vi "Test phi_offset Cpp.vi"() -> ()   [LabVIEW 2011]
uses:
  gVision.lvlib
panel:
  in  "yaw":dbl
  in  "roll":dbl
  in  "pitch":dbl
  out "phi":dbl
  out "error out":errorcluster
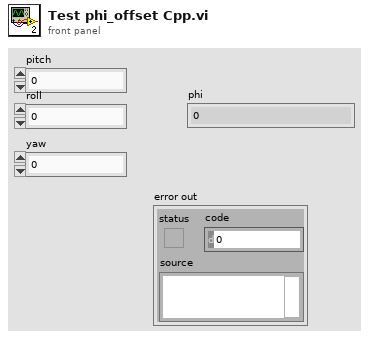
[diagram p1: front panel]
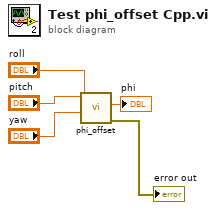
[diagram p0: block diagram]
diagram:
  n1 = call "phi_offset.vi"("yaw"="yaw", "roll"="roll", "pitch"="pitch") -> ("error out"=→"error out":errorcluster, "phi"=→"phi":dbl)  [unwired: 7 in]
